vi "Init GPS.vi"() -> (3 "Cluster":T1)   [LabVIEW 2013]
uses:
  Data/TypeDefs/GPS-Compass Queue Cluster.ctl
  Data/TypeDefs/GPS Sensor Status.ctl
  Data/TypeDefs/UTM Location.ctl
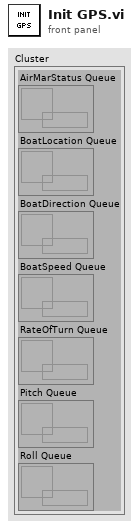
[diagram p1: front panel]
types:
  T1 = typedef "GPS-Compass Queue Cluster.ctl" = cluster{"AirMarStatus Queue":refnum<queue>, "BoatLocation Queue":refnum<queue>, "BoatDirection Queue":refnum<queue>, "BoatSpeed Queue":refnum<queue>, "RateOfTurn Queue":refnum<queue>, "Pitch Queue":refnum<queue>, "Roll Queue":refnum<queue>}
  T2 = typedef "GPS Sensor Status.ctl" = cluster{"Sensor Connected":bool, "Sensor OK":bool, "GPS Lock":bool, "Sensor Initialized":bool}
  T3 = typedef "UTM Location.ctl" = cluster{"UTM Zone":dbl, "Hemisphere":enum16{"North", "South"}, "East":dbl, "North":dbl}
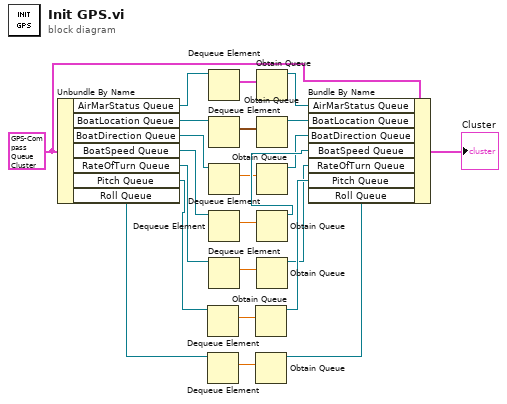
[diagram p0: block diagram]
diagram:
  w1 = T1 {"AirMarStatus Queue"=refnum, "BoatLocation Queue"=refnum, "BoatDirection Queue"=refnum, "BoatSpeed Queue"=refnum, "RateOfTurn Queue"=refnum, "Pitch Queue"=refnum, "Roll Queue"=refnum}
  n1 = Unbundle By Name(w1) -> ("AirMarStatus Queue"=w2:refnum<queue>, "BoatLocation Queue"=w5:refnum<queue>, "BoatDirection Queue"=w10:refnum<queue>, "BoatSpeed Queue"=w11:refnum<queue>, "RateOfTurn Queue"=w14:refnum<queue>, "Pitch Queue"=w19:refnum<queue>, "Roll Queue"=w22:refnum<queue>)
  n2 = Dequeue Element(queue=w19) -> (element=w18:dbl)  [unwired: 2 in, 3 out]
  n3 = Dequeue Element(queue=w22) -> (element=w17:dbl)  [unwired: 2 in, 3 out]
  n4 = Dequeue Element(queue=w2) -> (element=w3:T2)  [unwired: 2 in, 3 out]
  n5 = Dequeue Element(queue=w5) -> (element=w6:T3)  [unwired: 2 in, 3 out]
  n6 = Dequeue Element(queue=w10) -> (element=w9:dbl)  [unwired: 2 in, 3 out]
  n7 = Dequeue Element(queue=w11) -> (element=w12:dbl)  [unwired: 2 in, 3 out]
  n8 = Dequeue Element(queue=w14) -> (element=w13:dbl)  [unwired: 2 in, 3 out]
  n9 = Obtain Queue ("AirmarGPS-Compass Queue")(element data type=w18) -> (queue out=w20:refnum<queue>)  [unwired: 4 in, 2 out]
  n10 = Obtain Queue ("AirmarGPS-Compass Queue")(element data type=w17) -> (queue out=w21:refnum<queue>)  [unwired: 4 in, 2 out]
  n11 = Obtain Queue ("AirmarGPS-Compass Queue")(element data type=w3) -> (queue out=w4:refnum<queue>)  [unwired: 4 in, 2 out]
  n12 = Obtain Queue ("AirmarGPS-Compass Queue")(element data type=w6) -> (queue out=w7:refnum<queue>)  [unwired: 4 in, 2 out]
  n13 = Obtain Queue ("AirmarGPS-Compass Queue")(element data type=w9) -> (queue out=w8:refnum<queue>)  [unwired: 4 in, 2 out]
  n14 = Obtain Queue ("AirmarGPS-Compass Queue")(element data type=w12) -> (queue out=w16:refnum<queue>)  [unwired: 4 in, 2 out]
  n15 = Obtain Queue ("AirmarGPS-Compass Queue")(element data type=w13) -> (queue out=w15:refnum<queue>)  [unwired: 4 in, 2 out]
  n16 = Bundle By Name(cluster=w1, "AirMarStatus Queue"=w4, "BoatLocation Queue"=w7, "BoatDirection Queue"=w8, "BoatSpeed Queue"=w16, "RateOfTurn Queue"=w15, "Pitch Queue"=w20, "Roll Queue"=w21) -> (→"Cluster":T1)
